vi "Read.vi"(7 "I2C Channel (0)":u8, 8 "Error In":errorcluster, 9 "Resolution":enum16{"2g", "4g", "8g", "16g"}(ring), 10 "I2C Slave Address":T8, 11 "LINX Resource":T1) -> (0 "Error Out":errorcluster, 2 "Acceleration Data (g)":T7, 3 "LINX Resource":T1)   [LabVIEW 2020, in "LMH-LINX.lvlib" / "PmodACL.lvlib"]
doc: "Read acceleration data (in g's) from the PmodACL."
uses:
  PmodACL.lvlib
  Accelerometer/ADXL345/Address.ctl
  Private/Type Defs/LINX Ref.ctl
  Private/Type Defs/Platform.ctl
  Private/Type Defs/Interface.ctl
  Private/Device/Type Defs/LINX Device Config.ctl
  Private/Device/Type Defs/TCP Config.ctl
  Private/Device/Type Defs/Channels.ctl
  Accelerometer/ADXL345/ADXL345.lvlib
  LMH-LINX.lvlib
  Private/Device/Device.lvlib
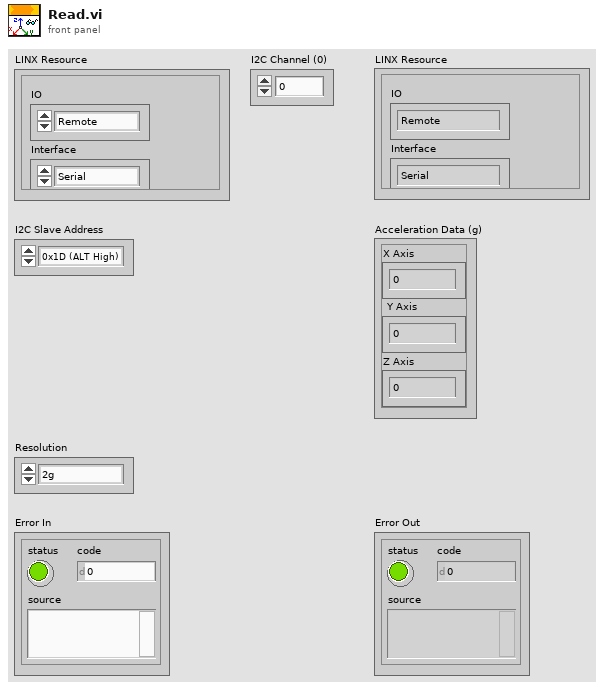
[diagram p1: front panel]
types:
  T1 = typedef "LMH-LINX.lvlib/LINX Ref.ctl" = cluster{"IO":T2, "Interface":T3, "LINX Device Config":T4}
  T2 = typedef "LMH-LINX.lvlib/Platform.ctl" = enum16{"Remote", "Local"}
  T3 = typedef "LMH-LINX.lvlib/Interface.ctl" = enum16{"Serial", "TCP"}
  T4 = typedef "LMH-LINX.lvlib/Device.lvlib/LINX Device Config.ctl" = cluster{"Interface":T3, "COM Port":refnum<visa-resource-name>, "TCP Configuration":T5, "Device Family":u8, "Device ID":u8, "Device Name":string, "TCP Ref":refnum<k5>, "Channels":T6}
  T5 = typedef "LMH-LINX.lvlib/Device.lvlib/TCP Config.ctl" = cluster{"IP Address":string, "Port":u16}
  T6 = typedef "LMH-LINX.lvlib/Channels.ctl" = cluster{"DI":u8[], "DO":u8[], "AI":u8[], "AO":u8[], "PWM":u8[], "QE":u8[], "UART":u8[], "I2C 2":u8[], "SPI":u8[], "CAN":u8[], "Servo":u8[], "AI Ref (V)":dbl, "AI Resolution (Bits)":u8, "AO Ref (V)":dbl, "AO Resolution (Bits)":u8}
  T7 = cluster{"X Axis":dbl, "Y Axis":dbl, "Z Axis":dbl}
  T8 = typedef "LMH-LINX.lvlib/ADXL345.lvlib/Address.ctl" = enum16{"0x1D (ALT High)", "0x53 (ALT Low)"}
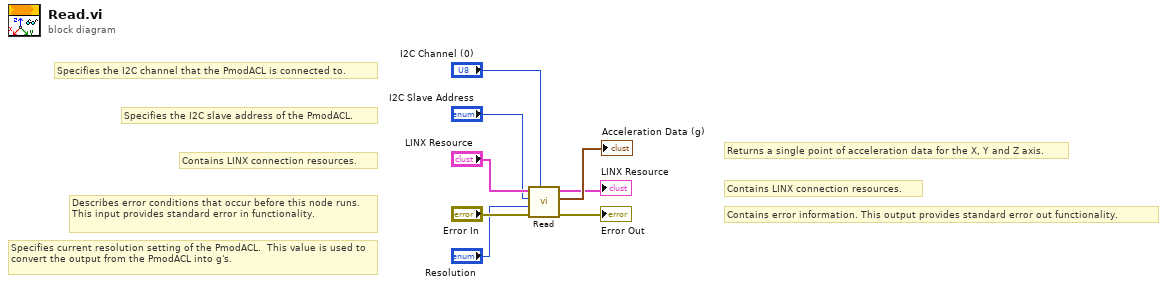
[diagram p0: block diagram]
diagram:
  # "Returns a single point of acceleration data for the X, Y and Z axis."
  # "Contains LINX connection resources."
  # "Contains error information. This output provides standard error out functionality."
  # "Specifies current resolution setting of the PmodACL.  This value is used to convert the output from the PmodACL into g's."
  # "Specifies the I2C slave address of the PmodACL."
  # "Specifies the I2C channel that the PmodACL is connected to."
  # "Contains LINX connection resources."
  # "Describes error conditions that occur before this node runs. This input provides standard error in functionality."
  n1 = call "Read.vi"("I2C Channel (0)"="I2C Channel (0)", "Error In"="Error In", "Resolution"="Resolution", "I2C Slave Address"="I2C Slave Address", "LINX Resource"="LINX Resource") -> ("Error Out"=→"Error Out":errorcluster, "Acceleration Data (g)"=→"Acceleration Data (g)":T7, "LINX Resource"=→"LINX Resource":T1)  [unwired: 4 in]
